vi "Wave Memory write from DMA - Host.vi"(8 "error in":errorcluster, 11 "FPGA VI Reference In":refnum<k20>) -> (0 "FPGA VI Reference Out":refnum<k20>, 3 "error out":errorcluster, 6 "Write memory complete":bool)   [LabVIEW 2014]
uses:
  <vilib>/rvi/interface/common/niFpgaWaitOnOcc.vi
  <vilib>/Utility/error.llb/Error Cluster From Error Code.vi
  <vilib>/rvi/errors/niLvFpgaAdjustHostInterfaceError.vi
  <vilib>/RVI Host/nirviSupport.llb/nirviErrorClusterFromErrorCode.vi
  <vilib>/rvi/interface/nirviMethod/nirviMethod.xnode
  <vilib>/rvi/errors/niLvFpgaMergeErrorWithErrorCode.vi
  <vilib>/rvi/interface/nirviMethod/StockFPGA_InlinedMethodWaitForSingleIRQ.vi
  <vilib>/FPGAPlugInAG/Dynamic/niLvFpga_WaitOnIrq_Dynamic.vi
  <vilib>/FPGAPlugInAG/Dynamic/niLvFpga_AcknowledgeIrq_Dynamic.vi
  <vilib>/FPGAPlugInAG/Dynamic/niLvFpga_ConfigureFifo_Dynamic.vi
  <vilib>/FPGAPlugInAG/Dynamic/niLvFpga_StartFifo_Dynamic.vi
  <vilib>/FPGAPlugInAG/Dynamic/niLvFpga_WriteFifo_Dynamic.vi
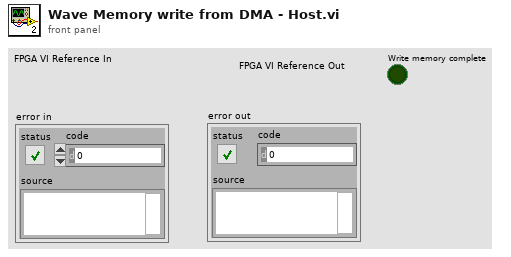
[diagram p1: front panel]
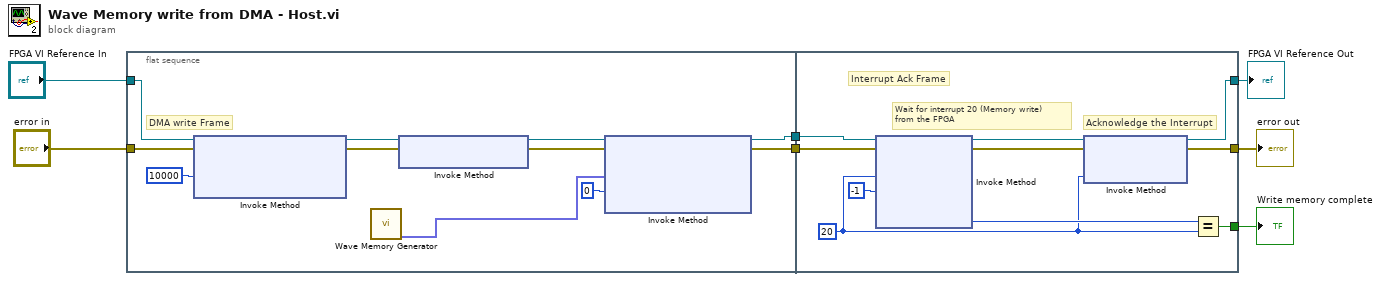
[diagram p0: block diagram]
diagram:
  n1 = flat-sequence {
    tunnel: [w12] -> w7
    tunnel: [w11] -> w6
    tunnel: "error in" -> [w10]
    tunnel: "FPGA VI Reference In" -> [w9]
    tunnel: [w22] -> w1
    tunnel: [w23] -> w5
    tunnel: w7 -> [w27]
    tunnel: w6 -> [w28]
    tunnel: [w19] -> w4
    frame #0 {
      # "DMA write Frame"
      n2 = xnode "Invoke Method"("FPGA VI Reference In"=w9, "error in"=w10, "Requested Depth"=u32 10000) -> ("FPGA VI Reference Out"=w17:refnum<k20>, "error out"=w16:errorcluster)  [unwired: 1 out]
      n3 = call "Wave Memory Generator.vi"() -> ("FXP Init Data Out"=w8:fxp<+/-,12,12>[])  [unwired: 10 in, 1 out]
      n4 = xnode "Invoke Method"("FPGA VI Reference In"=w17, "error in"=w16) -> ("FPGA VI Reference Out"=w14:refnum<k20>, "error out"=w15:errorcluster)
      n5 = xnode "Invoke Method"("FPGA VI Reference In"=w14, "error in"=w15, "Data"=w8, "Timeout (ms)"=0) -> ("FPGA VI Reference Out"=w12:refnum<k20>, "error out"=w11:errorcluster)  [unwired: 1 out]
    }
    frame #1 {
      w20 = 20 ("IRQ Number(s)")
      # "Acknowledge the Interrupt"
      # "Wait for interrupt 20 (Memory write)\nfrom the FPGA"
      # "Interrupt Ack Frame"
      n6 = xnode "Invoke Method"("FPGA VI Reference In"=w27, "error in"=w28, "IRQ Number(s)"=w20, "Timeout (ms)"=-1) -> ("FPGA VI Reference Out"=w24:refnum<k20>, "error out"=w25:errorcluster, "IRQ(s) Asserted"=w21:i32)  [unwired: 1 out]
      n7 = xnode "Invoke Method"("FPGA VI Reference In"=w24, "error in"=w25, "IRQ Number(s)"=w20) -> ("FPGA VI Reference Out"=w22:refnum<k20>, "error out"=w23:errorcluster)
      n8 = Equal?(x=w21, y=w20) -> (x = y?=w19:bool)
    }
  }
  "error out" <- w5
  "Write memory complete" <- w4
  "FPGA VI Reference Out" <- w1
